vi "Create Lossless Reader.vi"(7 "Depth (Unlimited)":i32=-1, 8 "error in (no error)":errorcluster, 11 "Enclave in":refnum<class "Enclave.lvclass">) -> (0 "error out":errorcluster, 2 "Lossless":refnum<class "Lossless.lvclass">, 3 "Enclave out":refnum<class "Enclave.lvclass">)   [LabVIEW 2022 SP3, in "Enclave.lvlib" / "Enclave.lvclass"]
uses:
  Enclave.lvclass
  Lossless/Lossless.lvclass
  Element.ctl
  Enclave.lvclass/Enclave.ctl
  Enclave.lvlib
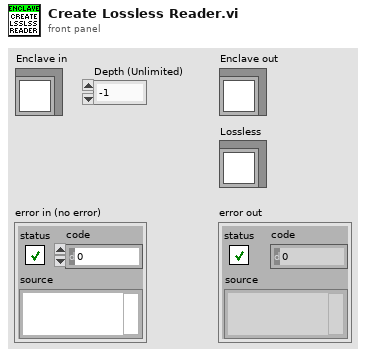
[diagram p1: front panel]
types:
  T1 = typedef "Enclave.lvlib/Element.ctl" = dbl
  T2 = typedef "Enclave.lvlib/Writer Data.ctl" = cluster{"Queues":refnum<queue>[], "Lossy":bool, "Event":bool}
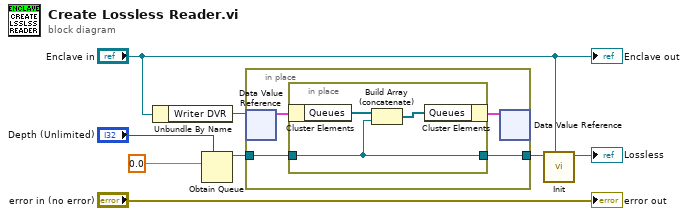
[diagram p0: block diagram]
diagram:
  n1 = Unbundle By Name("Enclave in") -> ("Writer DVR"=w7:refnum<data-value>)
  n2 = Obtain Queue(max queue size (-1, unlimited)="Depth (Unlimited)", element data type=T1 0.0 ("Element")) -> (queue out=w5:refnum<queue>)  [unwired: 3 in, 2 out]
  n3 = in-place {
    in-place-border: w5 -> [w11]
    in-place-border: [w9] -> w4
    n4 = in-place-dvr #1(w7) -> (w12:T2)  [unwired: 1 out]
    n5 = in-place {
      in-place-border: w11 -> [w13]
      in-place-border: [w13] -> w9
      n6 = in-place-cluster #2(w12) -> ("Queues"=w15:refnum<queue>[])
      n7 = Build Array (concatenate)(w15, w13) -> (w14:refnum<queue>[])
      n8 = in-place-cluster #2("Queues"=w14) -> (w10:T2)
    }
    n9 = in-place-dvr #1(w10) -> ()  [unwired: 2 out]
  }
  n10 = call "Init.vi"("Enclave"="Enclave in", "Queue"=w4) -> ("Lossless out"=→"Lossless":refnum<class "Lossless.lvclass">)  [unwired: 8 in, 1 out]
  "error out" <- "error in (no error)"
  "Enclave out" <- "Enclave in"
